vi "mail_number_upload_system_user.vi"() -> ()   [LabVIEW 2011]
doc: "This example opens a connection to a database specified by the Connection string (replace the DNS name with your database) inserts a new row into the table \"myOtherTable\" (replace the SQL string with your own SQL query)."
panel:
  in  "?":bool
  out "上傳結果：":string
  in  "輸入郵件編號":string
  # "退輔會 就學就業處 - 郵件編號上傳系統 v1.0"
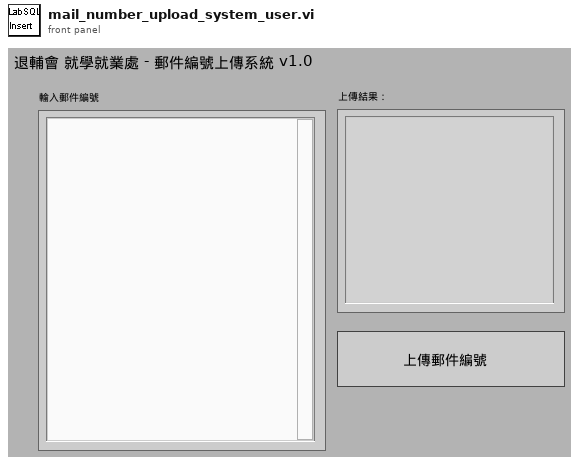
[diagram p1: front panel]
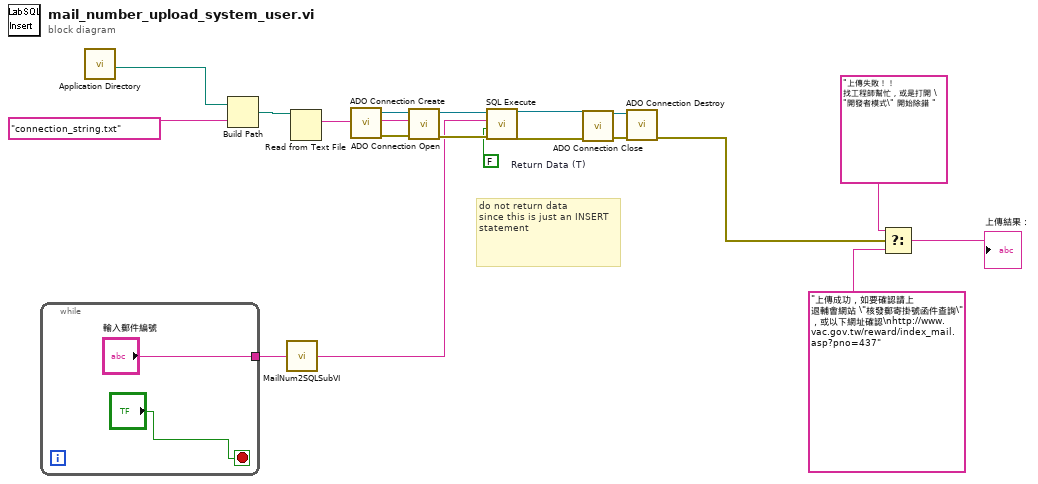
[diagram p0: block diagram]
diagram:
  w11 = FALSE  # Return Data (T)
  # "do not return data\nsince this is just an INSERT statement"
  n1 = while {
    tunnel: ["輸入郵件編號"] -> w10
    stop <- "?" stop-if-true
  }
  n2 = call <vilib>:"Application Directory.vi"() -> ("Application Directory"=w2:path)
  n3 = Build Path(base path=w2, name or relative path="connection_string.txt") -> (appended path=w3:path)
  n4 = call "MailNum2SQLSubVI.vi"("mail numbers"=w10) -> ("String"=w9:string)
  n5 = Read from Text File(file (use dialog)=w3) -> (text=w1:string)  [unwired: 3 in, 3 out]
  n6 = call "ADO Connection Create.vi"() -> ("error out"=w18:errorcluster, "ADODB._Connection Out"=w19:refnum<k7>)  [unwired: 10 in]
  n7 = call "ADO Connection Open.vi"("error in (no error)"=w18, "ConnectionString"=w1, "ADODB._Connection In"=w19) -> ("error out"=w16:errorcluster, "ADODB._Connection Out"=w17:refnum<k7>)  [unwired: 7 in]
  n8 = call "SQL Execute.vi"("error in (no error)"=w16, "Return Data (T)"=w11, "Command Text"=w9, "ADODB._Connection In"=w17) -> ("error out"=w15:errorcluster, "ADODB._Connection Out"=w14:refnum<k7>)  [unwired: 4 in, 2 out]
  n9 = call "ADO Connection Close.vi"("error in (no error)"=w15, "ADODB._Connection In"=w14) -> ("error out"=w13:errorcluster, "ADODB._Connection Out"=w12:refnum<k7>)  [unwired: 8 in]
  n10 = call "ADO Connection Destroy.vi"("error in (no error)"=w13, "ADODB._Connection In"=w12) -> ("error out"=w5:errorcluster)  [unwired: 9 in]
  n11 = Select(t="上傳失敗！！ 找工程師幫忙，或是打開 \"開發者模式\" 開始除錯 " ("f"), s=w5, f="上傳成功，如要確認請上 退輔會網站 \"核發郵寄掛號函件查詢\" ，或以下網址確認\nhttp://www.vac.gov.tw/reward/index_mail.asp?pno=437" ("上傳結果：")) -> (s? t:f=→"上傳結果：":string)
